vi "Disconnect_LCR.vi"(8 "error in (no error)":errorcluster, 10 "Parameters":string, 11 "reference in":refnum<class "Test_NanoP5.lvclass">) -> (0 "error out":errorcluster, 2 "Result":bool, 3 "reference out":refnum<class "Test_NanoP5.lvclass">)   [LabVIEW 2019]
uses:
  Test_NanoP5.lvclass
  <vilib>/addons/_JKI.lib/Serialization/JSON/JKI JSON Serialization.lvlib
  Components/SwitchBase.lvlibp/SwitchBase.lvclass
  ParameterTypes/Connect_LCR.ctl
panel:
  in  "Parameter_Type":T1
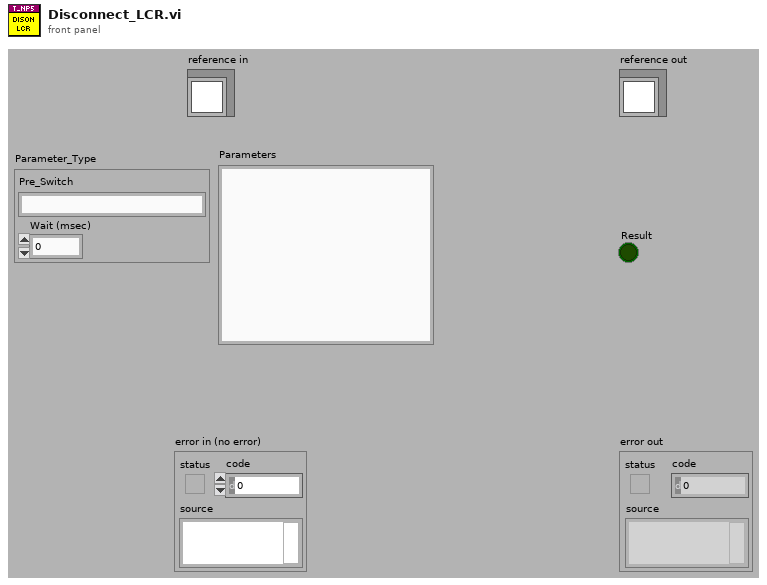
[diagram p1: front panel]
types:
  T1 = typedef "Test_NanoP5.lvlib/Test_NanoP5.lvclass/Connect_LCR.ctl" = cluster{"Pre_Switch":string, "Wait (msec)":i32}
  T2 = typedef "Test_NanoP5.lvlib/Test_NanoP5.lvclass/ObjectAttributes.ctl" = cluster{"Config":T3, "DMM":refnum<class "DMM_Keysight_34980A.lvclass">, "LCR":refnum<class "LCR_BK891.lvclass">, "PSU":refnum<class "PSU_Base.lvclass">, "Switch_Manager":refnum<class "SwitchBase.lvclass">, "Switch_Motor":refnum<class "SwitchBase.lvclass">, "NanoP5":refnum<class "NanoP5.lvclass">}
  T3 = typedef "Test_NanoP5.lvlib/Test_NanoP5.lvclass/Config.ctl" = cluster{"default":string}
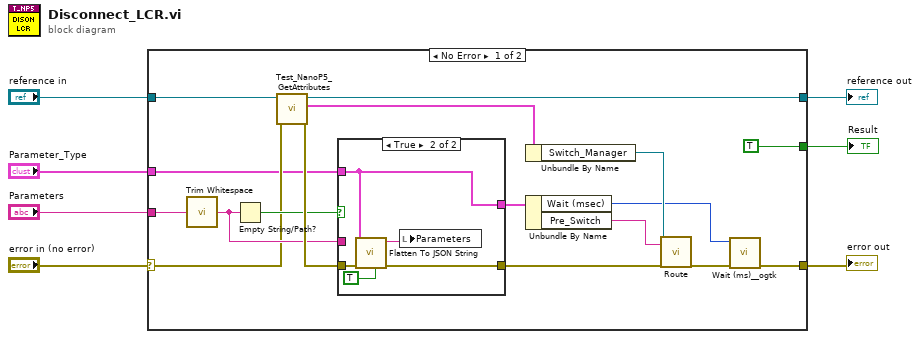
[diagram p0: block diagram]
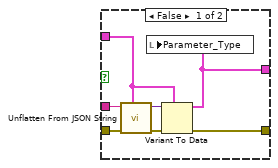
[diagram p2: hidden frame]
diagram:
  n1 = case shown="No Error" "error in (no error)" {
    selector: "error in (no error)" -> [w15 w38]
    tunnel: [w19 w38] -> w6
    tunnel: [w10 w37] -> w4
    tunnel: "reference in" -> [w13 w37]
    tunnel: "Parameters" -> [w11 _]
    tunnel: "Parameter_Type" -> [w12 _]
    tunnel: [TRUE _] -> w1
    frame No Error {
      n2 = call <vilib>:"Trim Whitespace.vi"("string"=w11) -> ("trimmed string"=w16:string)  [unwired: 1 in]
      n3 = Empty String/Path?(string/path=w16) -> (empty?=w17:bool)
      n4 = call "Test_NanoP5_GetAttributes.vi"("error in (no error)"=w15, "reference in"=w13) -> ("error out"=w18:errorcluster, "Data"=w9:T2, "reference out"=w10:refnum<class "Test_NanoP5.lvclass">)  [unwired: 6 in, 1 out]
      n5 = case shown="True" w17 {
        tunnel: w18 -> [w29 w35]
        tunnel: w12 -> [w28 w34]
        tunnel: [w27 w36] -> w14
        tunnel: [w25 w34] -> w8
        tunnel: w16 -> [w26 _]
        frame False {
          n6 = call <vilib>:"Unflatten From JSON String.vi"("Type and Defaults"=w28, "error in (no error)"=w29, "JSON String"=w26) -> ("error out"=w31:errorcluster, "Variant"=w30:variant)  [unwired: 7 in]
          n7 = Variant To Data(error in=w31, type=w28, Variant=w30) -> (data=w25:T1, error out=w27:errorcluster)
          n8 = local write "Parameter_Type"(w25) -> ()
        }
        frame True {
          n9 = call <vilib>:"Flatten To JSON String.vi"("Enums As String (F)"=TRUE, "error in (no error)"=w35, "Variant"=w34) -> ("error out"=w36:errorcluster, "JSON String"=w33:string)  [unwired: 7 in]
          n10 = local write "Parameters"(w33) -> ()
        }
      }
      n11 = Unbundle By Name(w9) -> ("Switch_Manager"=w24:refnum<class "SwitchBase.lvclass">)
      n12 = Unbundle By Name(w8) -> ("Wait (msec)"=w21:i32, "Pre_Switch"=w23:string)
      n13 = call-dynamic "Route.vi"("reference in"=w24, "channel 1"=w23, "error in (no error)"=w14) -> ("error out"=w22:errorcluster)  [unwired: 15 in, 1 out]
      n14 = call <userlib>:"Wait (ms)__ogtk.vi"("error in (no error)"=w22, "milliseconds to wait"=w21) -> ("error out"=w19:errorcluster)  [unwired: 8 in, 1 out]
    }
    frame Error {
    }
  }
  "Result" <- w1
  "error out" <- w6
  "reference out" <- w4
